vi "5011 Array Dimension Not Supported.vi"(8 "error in (no error)":errorcluster) -> (0 "error out":errorcluster)   [LabVIEW 2020, in "MacroAssert.lvlib" / "Custom Errors.lvlib"]
uses:
  Custom Errors.lvlib
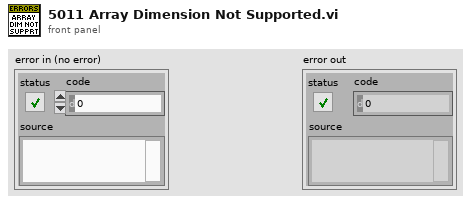
[diagram p1: front panel]
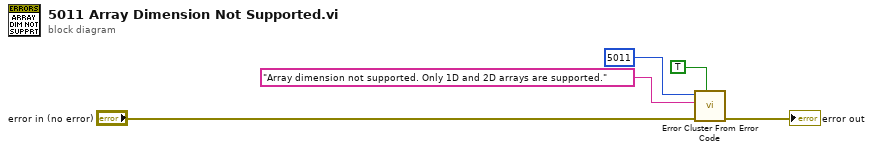
[diagram p0: block diagram]
diagram:
  n1 = call <vilib>:"Error Cluster From Error Code.vi"("show call chain? (False)"=TRUE, "error in (no error)"="error in (no error)", "error message (\"\")"="Array dimension not supported. Only 1D and 2D arrays are supported.", "error code (0)"=5011) -> ("error out"=→"error out":errorcluster)  [unwired: 5 in]
